vi "getWaypoints.vi"(8 "Error In":errorcluster, 11 "RoundBouy in":refnum<class "RoundBouy.lvclass">) -> (0 "Error Out":errorcluster, 2 "Waypoint Array":refnum<class "Waypoint.lvclass">[](array[class]), 3 "RoundBouy out":refnum<class "RoundBouy.lvclass">)   [LabVIEW 2013, in "RoundBouy.lvclass"]
uses:
  RoundBouy.lvclass
  Waypoint/Waypoint.lvclass
  Data/TypeDefs/UTM Location.ctl
  GenericMission/GenericMission.lvclass
  <vilib>/Analysis/baseanly.llb/Unit Vector (DBL).vi
  <vilib>/Analysis/coordinate.llb/2D Cartesian Coordinate Rotation (Scalar).vi
  <vilib>/Analysis/NI_AALBase.lvlib
  <vilib>/Analysis/NI_AALPro.lvlib
panel:
  in  "Next Mission Location":T1 {"North" format="%#_10f"; "East" format="%#_8f"}
  in  "Boats Current Position":T1 {"North" format="%#_10f"; "East" format="%#_8f"}
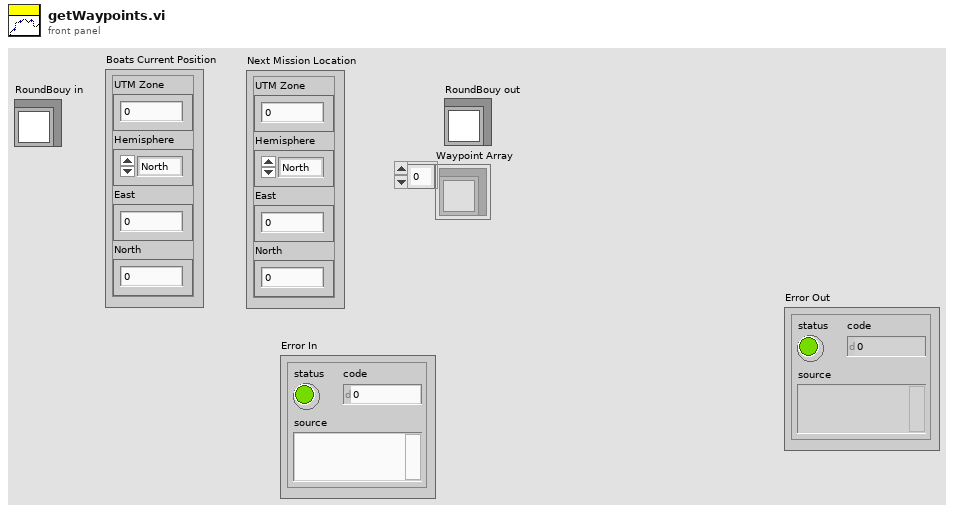
[diagram p1: front panel]
types:
  T1 = typedef "UTM Location.ctl" = cluster{"UTM Zone":dbl, "Hemisphere":enum16{"North", "South"}, "East":dbl, "North":dbl}
  T2 = typedef "MissionTypeControl.ctl" = enum16{"Idle at Point", "Drive to Waypoint", "Round Buoy to Port", "Round Buoy to Starboard", "Pass Between Buoys", "Station Keeping"}
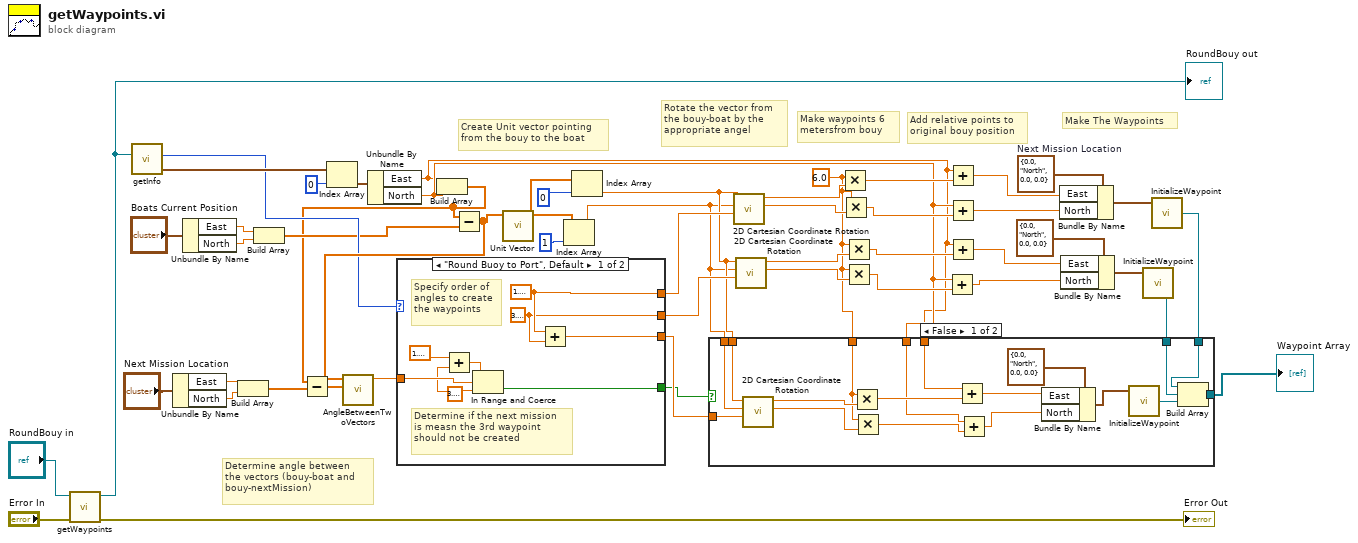
[diagram p0: block diagram]
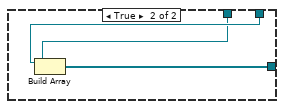
[diagram p2: hidden frame]
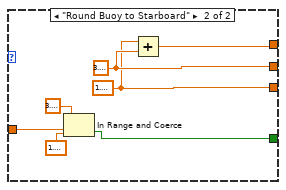
[diagram p3: hidden frame]
diagram:
  w32 = T1 {"UTM Zone"=0.0, "Hemisphere"=enum."North", "East"=0.0, "North"=0.0}  # Next Mission Location
  w9 = 6.0
  # "Create Unit vector pointing \nfrom the bouy to the boat"
  # "Determine angle between \nthe vectors (bouy-boat and \nbouy-nextMission)"
  # "Make The Waypoints"
  # "Rotate the vector from \nthe bouy-boat by the \nappropriate angel"
  # "Make waypoints 6 \nmetersfrom bouy"
  # "Add relative points to \noriginal bouy position"
  n1 = call-parent "getWaypoints.vi"("Error In"="Error In", "GenericMission in"="RoundBouy in") -> ("Error Out"=→"Error Out":errorcluster, "GenericMission out"=w48:refnum<class "RoundBouy.lvclass">)  [unwired: 7 in, 1 out]
  "RoundBouy out" <- w48
  n2 = call-dynamic "getInfo.vi"("GenericMission in"=w48) -> ("Points of Interest"=w16:T1[], "Mission Type"=w15:T2)  [unwired: 3 in, 6 out]
  n3 = Unbundle By Name("Next Mission Location") -> ("East"=w37:dbl, "North"=w38:dbl)
  n4 = Unbundle By Name("Boats Current Position") -> ("East"=w45:dbl, "North"=w44:dbl)
  n5 = Build Array(w37, w38) -> (w36:dbl[])
  n6 = Build Array(w45, w44) -> (w2:dbl[])
  n7 = Index Array(array=w16, index=0) -> (element=w46:T1)
  n8 = Unbundle By Name(w46) -> ("East"=w7:dbl, "North"=w8:dbl)
  n9 = Build Array(w7, w8) -> (w1:dbl[])
  n10 = Subtract(x=w1, y=w36) -> (x-y=w34:dbl[])
  n11 = Subtract(x=w1, y=w2) -> (x-y=w35:dbl[])
  n12 = call "AngleBetweenTwoVectors.vi"("Rotated Vector"=w34, "Base Vector"=w35) -> ("Angle Between Vectors"=w29:dbl)  [unwired: 9 in]
  n13 = case shown="\"Round Buoy to Port\", Default" w15 {
    tunnel: [w59 w65] -> w40
    tunnel: [w58 w66] -> w39
    tunnel: [w57 w64] -> w10
    tunnel: w29 -> [w56 w63]
    tunnel: [w55 w62] -> w3
    frame "Round Buoy to Port", Default {
      w53 = 3.141592653589793
      w58 = 3.141592653589793
      w59 = 1.5707963267948966
      # "Determine if the next mission \nis measn the 3rd waypoint \nshould not be created"
      # "Specify order of \nangles to create \nthe waypoints"
      n14 = Add(x=1.5707963267948966, y=w53) -> (x+y=w54:dbl)
      n15 = In Range and Coerce(upper limit=w54, x=w56, lower limit=w53) -> (In Range?=w55:bool)  [unwired: 1 out]
      n16 = Add(x=w59, y=w58) -> (x+y=w57:dbl)
    }
    frame "Round Buoy to Starboard" {
      w66 = 3.141592653589793
      w64 = 1.5707963267948966
      n17 = In Range and Coerce(upper limit=3.141592653589793, x=w63, lower limit=1.5707963267948966) -> (In Range?=w62:bool)  [unwired: 1 out]
      n18 = Add(x=w64, y=w66) -> (x+y=w65:dbl)
    }
  }
  n19 = call-poly <vilib>:"Unit Vector.vi"("Input Vector"=w35) -> ("Unit Vector"=w43:dbl[])  [unwired: 8 in, 2 out]
  n20 = Index Array(array=w43, index=1) -> (element=w11:dbl)
  n21 = Index Array(array=w43, index=0) -> (element=w12:dbl)
  n22 = call-poly <vilib>:"2D Cartesian Coordinate Rotation.vi"("theta"=w40, "y"=w11, "x"=w12) -> ("y out"=w27:dbl, "x out"=w28:dbl)  [unwired: 6 in, 1 out]
  n23 = call-poly <vilib>:"2D Cartesian Coordinate Rotation.vi"("theta"=w39, "y"=w11, "x"=w12) -> ("y out"=w26:dbl, "x out"=w25:dbl)  [unwired: 6 in, 1 out]
  n24 = Multiply(x=w9, y=w28) -> (x*y=w22:dbl)
  n25 = Multiply(x=w9, y=w27) -> (x*y=w21:dbl)
  n26 = Multiply(x=w9, y=w25) -> (x*y=w20:dbl)
  n27 = Multiply(x=w9, y=w26) -> (x*y=w19:dbl)
  n28 = Add(x=w8, y=w19) -> (x+y=w18:dbl)
  n29 = Add(x=w7, y=w22) -> (x+y=w23:dbl)
  n30 = Add(x=w8, y=w21) -> (x+y=w24:dbl)
  n31 = Add(x=w7, y=w20) -> (x+y=w17:dbl)
  n32 = Bundle By Name(cluster=w32, "East"=w23, "North"=w24) -> (w33:T1)
  n33 = Bundle By Name(cluster=T1 {"UTM Zone"=0.0, "Hemisphere"=enum."North", "East"=0.0, "North"=0.0} ("Next Mission Location"), "East"=w17, "North"=w18) -> (w30:T1)
  n34 = call "InitializeWaypoint.vi"("Coords"=w30) -> ("Waypoint Out"=w6:refnum<class "Waypoint.lvclass">)  [unwired: 2 in]
  n35 = call "InitializeWaypoint.vi"("Coords"=w33) -> ("Waypoint Out"=w5:refnum<class "Waypoint.lvclass">)  [unwired: 2 in]
  n36 = case shown="False" w3 {
    tunnel: [w84 w85] -> w4
    tunnel: w5 -> [w83 w87]
    tunnel: w6 -> [w82 w86]
    tunnel: w10 -> [w78 _]
    tunnel: w12 -> [w77 _]
    tunnel: w11 -> [w76 _]
    tunnel: w9 -> [w73 _]
    tunnel: w7 -> [w68 _]
    tunnel: w8 -> [w67 _]
    frame False {
      n37 = call-poly <vilib>:"2D Cartesian Coordinate Rotation.vi"("theta"=w78, "y"=w76, "x"=w77) -> ("y out"=w75:dbl, "x out"=w74:dbl)  [unwired: 6 in, 1 out]
      n38 = Multiply(x=w73, y=w74) -> (x*y=w69:dbl)
      n39 = Multiply(x=w73, y=w75) -> (x*y=w70:dbl)
      n40 = Add(x=w68, y=w69) -> (x+y=w71:dbl)
      n41 = Add(x=w67, y=w70) -> (x+y=w72:dbl)
      n42 = Bundle By Name(cluster=T1 {"UTM Zone"=0.0, "Hemisphere"=enum."North", "East"=0.0, "North"=0.0} ("Next Mission Location"), "East"=w71, "North"=w72) -> (w81:T1)
      n43 = call "InitializeWaypoint.vi"("Coords"=w81) -> ("Waypoint Out"=w79:refnum<class "Waypoint.lvclass">)  [unwired: 2 in]
      n44 = Build Array(w83, w82, w79) -> (w84:refnum<class "Waypoint.lvclass">[])
    }
    frame True {
      n45 = Build Array(w87, w86) -> (w85:refnum<class "Waypoint.lvclass">[])
    }
  }
  "Waypoint Array" <- w4
